vi "2DMain.vi"() -> ()   [LabVIEW 2016]
panel:
  out "XY Graph":cluster{dbl[], dbl[]}(graph)
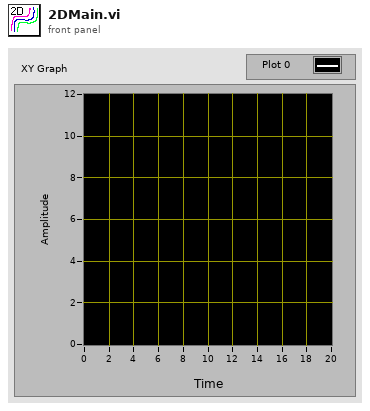
[diagram p1: front panel]
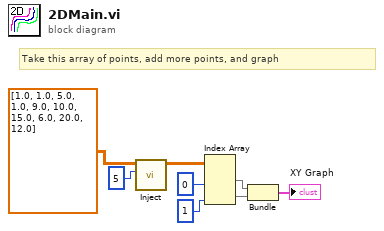
[diagram p0: block diagram]
diagram:
  # "Take this array of points, add more points, and graph"
  n1 = call "Inject.vi"("NumToInject"=5, "Array In"=dbl[][] [[1.0, 1.0], [5.0, 1.0], [9.0, 10.0], [15.0, 6.0], [20.0, 12.0]] ("transposed array")) -> ("Array Out"=w1:dbl[][])  [unwired: 9 in]
  n2 = Index Array(array=w1, index (col) #1=0 ("disabled index (col)"), index (col) #2=1 ("index (col)")) -> (element #1=w7:dbl[], element #2=w6:dbl[])  [unwired: 2 in]
  n3 = Bundle("Array Out"=w7, "Array Out"=w6) -> (→"XY Graph":cluster{"Array Out":dbl[], "Array Out":dbl[]})  [unwired: 1 in]
